vi "LaserCal-Save Data (PT).vi"(0 "System ID":T2, 7 "I-O Data":T3, 9 "Options":T1, 11 "error in (no error)":errorcluster) -> (15 "error out":errorcluster)   [LabVIEW 2015]
uses:
  Typedefs/LaserCal-Data (PT).ctl
  Typedefs/LaserCal-System ID.ctl
  Typedefs/LaserCal-Options.ctl
panel:
  in  "Laser Pulse Train Calibration File":T4
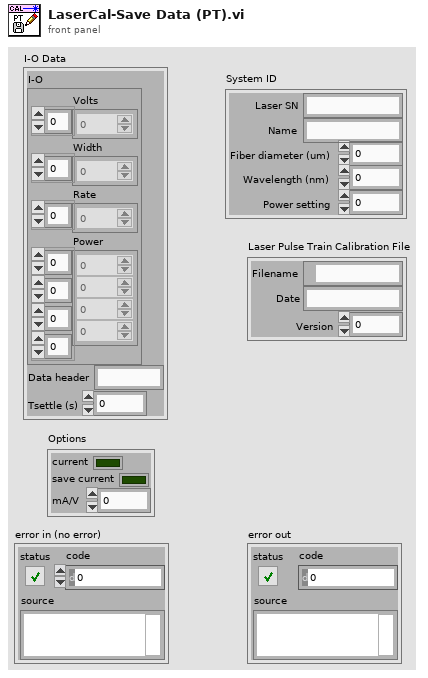
[diagram p1: front panel]
types:
  T1 = typedef "LaserCal-Options.ctl" = cluster{"current":bool, "save current":bool, "mA/V":dbl}
  T2 = typedef "LaserCal-System ID.ctl" = cluster{"Name":string, "Laser SN":string, "Wavelength (nm)":dbl, "Fiber diameter (um)":dbl, "Power setting":dbl}
  T3 = typedef "LaserCal-Data (PT).ctl" = cluster{"I-O":cluster{"Volts":dbl[], "Width":dbl[], "Rate":dbl[], "Power":dbl[][][][]}, "Data header":string, "Tsettle (s)":dbl}
  T4 = cluster{"Filename":path, "Date":string, "Version":i32}
  T5 = cluster{"Volts":dbl[], "Width":dbl[], "Rate":dbl[], "Power":dbl[][][][]}
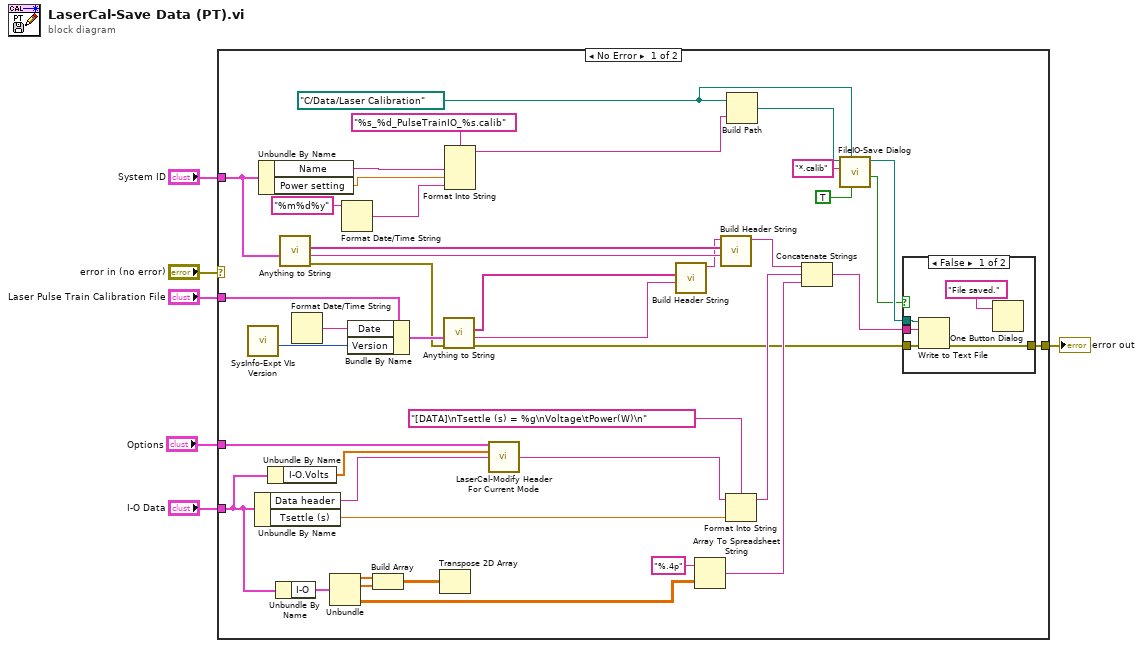
[diagram p0: block diagram]
diagram:
  n1 = case shown="No Error" "error in (no error)" {
    selector: "error in (no error)" -> [_ w55]
    tunnel: [w25 w55] -> w6
    tunnel: "Laser Pulse Train Calibration File" -> [w46 _]
    tunnel: "I-O Data" -> [w9 _]
    tunnel: "System ID" -> [w29 _]
    tunnel: "Options" -> [w12 _]
    frame No Error {
      w23 = path "C:/Data/Laser Calibration"
      n2 = call "SysInfo-Expt VIs Version.vi"() -> ("Expt VIs Version out"=w47:i32)  [unwired: 11 in]
      n3 = Unbundle By Name(w9) -> ("Data header"=w11:string, "Tsettle (s)"=w37:dbl)
      n4 = Unbundle By Name(w29) -> ("Name"=w28:string, "Power setting"=w18:dbl)
      n5 = Unbundle By Name(w9) -> ("I-O.Volts"=w8:dbl[])
      n6 = Unbundle By Name(w9) -> ("I-O"=w43:T5)
      n7 = call "Anything to String.vi"("Anything"=w29) -> ("Error Out"=w33:errorcluster, "Section"=w34:string, "Strings[]"=w32:string[])  [unwired: 8 in]
      n8 = Format Date/Time String() -> (date/time string=w48:string)  [unwired: 3 in]
      n9 = Unbundle(w43) -> ("Volts"=w42:dbl[], "Width"=w41:dbl[], "Power"=w15:dbl[][][][])  [unwired: 1 out]
      n10 = Format Date/Time String(time format string (%c)="%m%d%y") -> (date/time string=w16:string)  [unwired: 2 in]
      n11 = Bundle By Name(cluster=w46, "Date"=w48, "Version"=w47) -> (w45:T4)
      n12 = Build Array(w42, w41) -> (w40:dbl[][])
      n13 = Transpose 2D Array(2D array=w40) -> ()  [unwired: 1 out]
      n14 = call "Anything to String.vi"("Error In"=w33, "Anything"=w45) -> ("Error Out"=w22:errorcluster, "Section"=w10:string, "Strings[]"=w44:string[])  [unwired: 7 in]
      n15 = Format Into String(format string="%s_%d_PulseTrainIO_%s.calib", w28, w18, w16) -> (resulting string=w26:string)  [unwired: 2 in, 1 out]
      n16 = call "LaserCal-Modify Header For Current Mode.vi"("Options"=w12, "Volts"=w8, "header in"=w11) -> ("header out"=w7:string)  [unwired: 12 in]
      n17 = call "Build Header String.vi"("Section"=w10, "Strings[]"=w44) -> ("Header out"=w31:string)  [unwired: 9 in]
      n18 = Array To Spreadsheet String(array=w15, 3:"%.4p" ("format string")) -> (spreadsheet string=w35:string)  [unwired: 1 in]
      n19 = call "Build Header String.vi"("Section"=w34, "Strings[]"=w32, "Header in"=w31) -> ("Header out"=w30:string)  [unwired: 8 in]
      n20 = Format Into String(format string="[DATA]\nTsettle (s) = %g\nVoltage\tPower(W)\n", initial string=w7, w37) -> (resulting string=w36:string)  [unwired: 1 in, 1 out]
      n21 = Build Path(base path=w23, name or relative path=w26) -> (appended path=w14:path)
      n22 = Concatenate Strings(w30, w36, w35) -> (w24:string)
      n23 = call "FileIO-Save Dialog.vi"("Overwrite prompt?"=TRUE, "Default Folder"=w23, "pattern (all files)"="*.calib", "Start path"=w14) -> ("cancelled"=w20:bool, "selected path"=w21:path)  [unwired: 5 in, 1 out]
      n24 = case shown="False" w20 {
        tunnel: [w53 w54] -> w25
        tunnel: w24 -> [w52 _]
        tunnel: w22 -> [w51 w54]
        tunnel: w21 -> [w50 _]
        frame False {
          n25 = Write to Text File(file (use dialog)=w50, text=w52, error in=w51) -> (error out=w53:errorcluster)  [unwired: 1 in, 2 out]
          n26 = One Button Dialog(message="File saved.") -> ()  [unwired: 1 in, 1 out]
        }
        frame True {
        }
      }
    }
    frame Error {
    }
  }
  "error out" <- w6
